vi "Get Test Suites.vi"(8 "error in (no error)":errorcluster) -> (0 "error out":errorcluster, 2 "Tests":refnum<class "Test.lvclass">[](array[class]))   [LabVIEW 2017, in "Test Explorer.lvlib"]
doc: "Returns a list of test suites from the current project.\n\n- Test libraries must be at the top-level inside the project (sublibraries will be ignored)\n- Test library names must end with \"Test.lvlib\""
uses:
  Test Explorer.lvlib
  Test/Test.lvclass
  TestBuilder/TestBuilder.lvclass
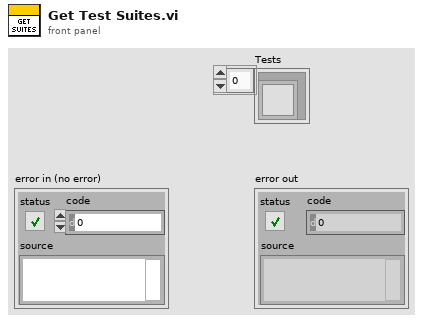
[diagram p1: front panel]
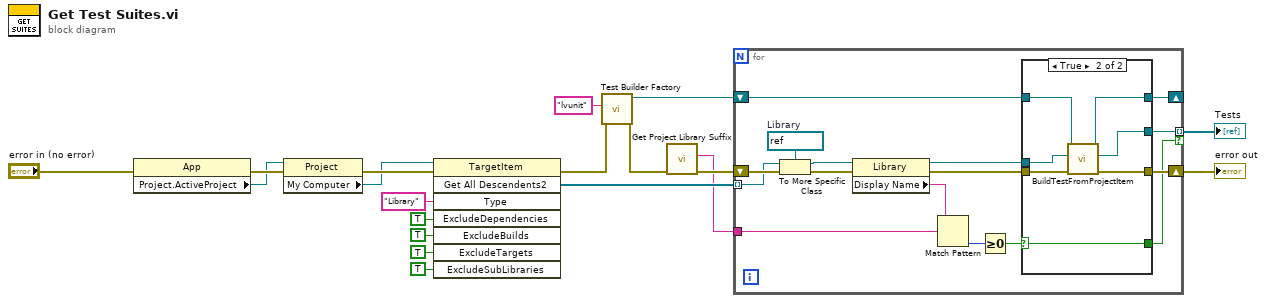
[diagram p0: block diagram]
diagram:
  n1 = property class="App"(error in="error in (no error)") -> (error out=w9:errorcluster, "Project.ActiveProject"=w7:refnum<vi>)  [unwired: 1 in, 1 out]
  n2 = property class="Project"(reference=w7, error in=w9) -> (error out=w19:errorcluster, "My Computer"=w12:refnum<vi>)  [unwired: 1 out]
  n3 = invoke class="TargetItem" method="Get All Descendents2"(reference=w12, error in=w19, "Type"="Library", "ExcludeDependencies"=TRUE, "ExcludeBuilds"=TRUE, "ExcludeTargets"=TRUE, "ExcludeSubLibraries"=TRUE) -> (error out=w5:errorcluster, "Get All Descendents2"=w14:refnum<vi>[])  [unwired: 1 in, 6 out]
  n4 = call "Test Builder Factory.vi"("error in (no error)"=w5, "Name"="lvunit") -> ("error out"=w3:errorcluster, "Test Builder"=w6:refnum<class "TestBuilder.lvclass">)  [unwired: 8 in]
  n5 = call "Get Project Library Suffix.vi"("error in (no error)"=w3) -> ("error out"=w2:errorcluster, "Project Library Suffix"=w1:string)  [unwired: 9 in]
  n6 = for {
    tunnel: w14 -> [w31] mode=indexing
    shift-right: [w28] -> w11
    shift-left: w2 -> [w33]
    tunnel: [w26] -> w10 mode=indexing if=w25
    shift-right: [w23] -> _
    shift-left: w6 -> [w22]
    tunnel: w1 -> [w21]
    w30 = refnum<vi> refnum  # Library
    n7 = To More Specific Class(target class=w30, reference=w31, error in=w33) -> (specific class reference=w20:refnum<vi>, error out=w32:errorcluster)
    n8 = property class="Library"(reference=w20, error in=w32) -> (reference out=w24:refnum<vi>, error out=w29:errorcluster, "Display Name"=w34:string)
    n9 = Match Pattern(string=w34, regular expression=w21) -> (offset past match=w35:i32)  [unwired: 1 in, 3 out]
    n10 = Greater Or Equal To 0?(x=w35) -> (x >= 0?=w27:bool)
    n11 = case shown="True" w27 {
      selector: w27 -> [w37 w45]
      tunnel: w29 -> [w38 w44]
      tunnel: [w38 w42] -> w28
      tunnel: [_ w41] -> w26
      tunnel: [w37 w45] -> w25
      tunnel: w24 -> [_ w43]
      tunnel: [w36 w40] -> w23
      tunnel: w22 -> [w36 w39]
      frame False {
      }
      frame True {
        n12 = call-dynamic "BuildTestFromProjectItem.vi"("error in (no error)"=w44, "ProjectItem Refnum"=w43, "TestBuilder in"=w39) -> ("error out"=w42:errorcluster, "Test"=w41:refnum<class "Test.lvclass">, "TestBuilder out"=w40:refnum<class "TestBuilder.lvclass">)  [unwired: 6 in]
      }
    }
  }
  "error out" <- w11
  "Tests" <- w10
